vi "WLAN - TV - RW - UTIL - CenterFrequencyToChannelNumber_bc.vi"(0 "Center Frequency(Hz)":dbl=4940000000.0, 5 "Channel Bandwidth (Hz)":dbl=20000000.0) -> (4 "Coherced Channel Number":i32=188, 6 "Coherced Center Frequency (Hz)":dbl=5180000000.0)   [LabVIEW 2012]
doc: "Return channe numer according to channel bandwidth and center frequency."
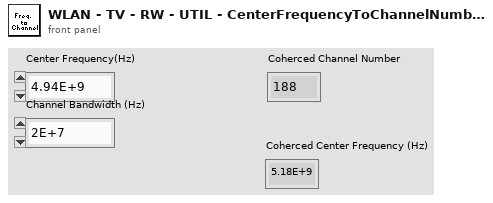
[diagram p1: front panel]
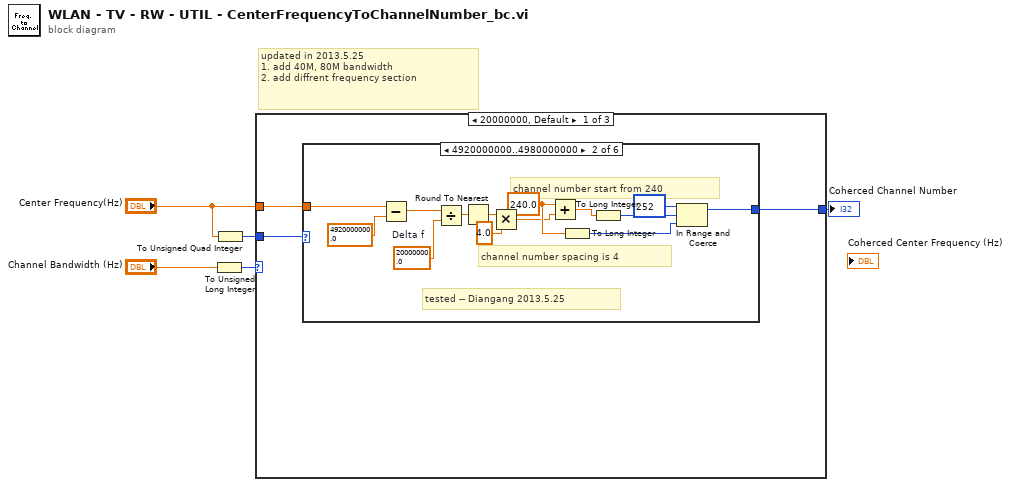
[diagram p0: block diagram]
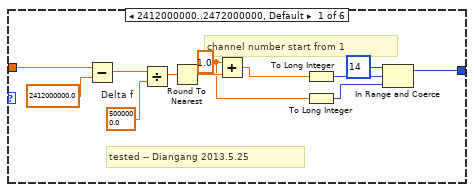
[diagram p2: hidden frame]
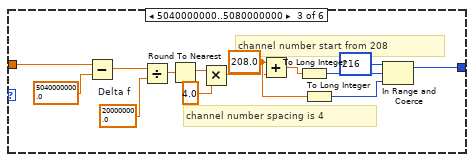
[diagram p3: hidden frame]
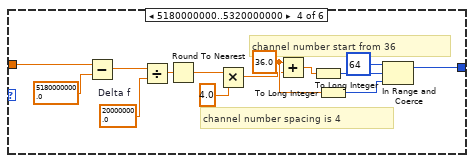
[diagram p4: hidden frame]
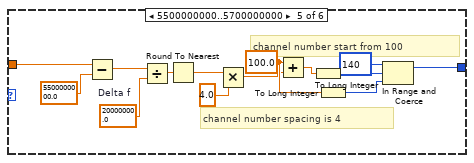
[diagram p5: hidden frame]
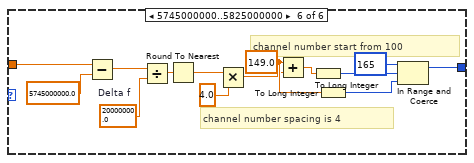
[diagram p6: hidden frame]
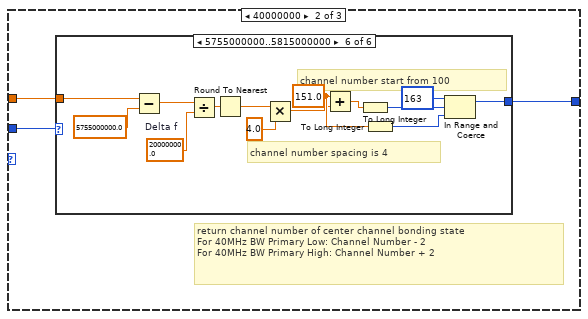
[diagram p7: hidden frame]
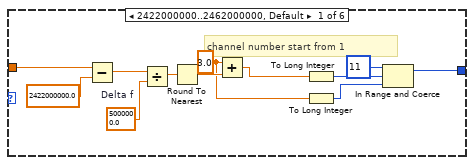
[diagram p8: hidden frame]
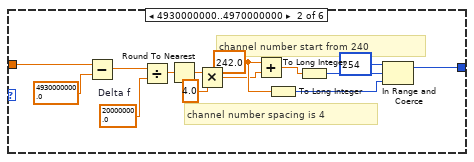
[diagram p9: hidden frame]
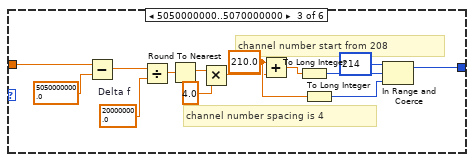
[diagram p10: hidden frame]
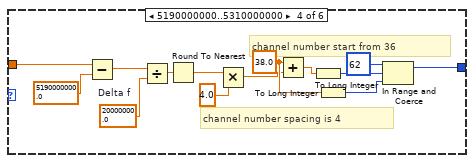
[diagram p11: hidden frame]
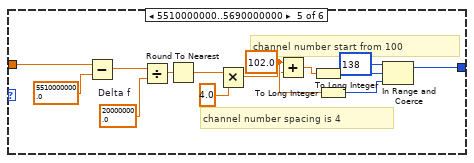
[diagram p12: hidden frame]
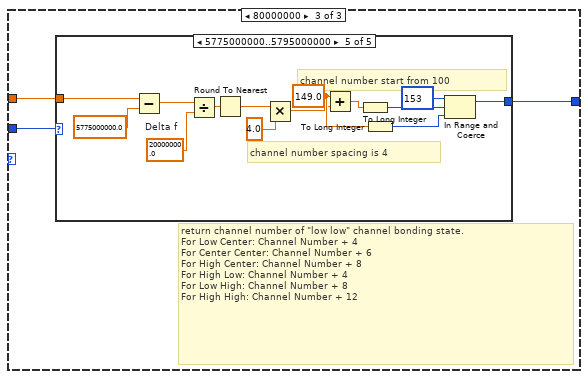
[diagram p13: hidden frame]
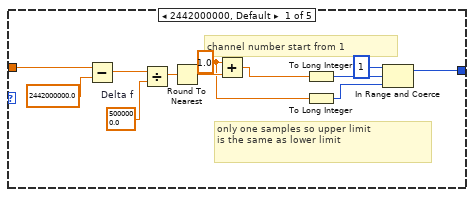
[diagram p14: hidden frame]
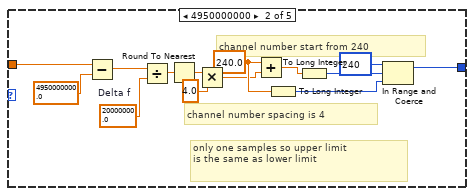
[diagram p15: hidden frame]
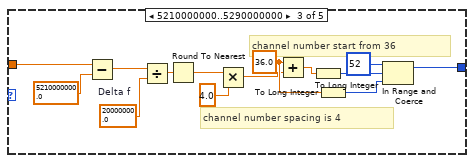
[diagram p16: hidden frame]
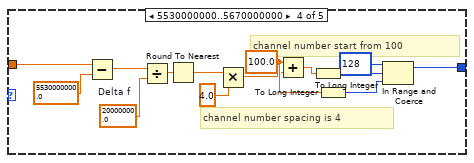
[diagram p17: hidden frame]
diagram:
  # "updated in 2013.5.25\n1. add 40M, 80M bandwidth\n2. add diffrent frequency section"
  n1 = To Unsigned Long Integer(number="Channel Bandwidth (Hz)") -> (unsigned 32bit integer=w4:u32)
  n2 = To Unsigned Quad Integer(1:"Center Frequency(Hz)") -> (0:w3:u64)
  n3 = case shown="20000000, Default" w4 {
    tunnel: w3 -> [w8 w93 w178]
    tunnel: "Center Frequency(Hz)" -> [w7 w92 w177]
    tunnel: [w6 w91 w176] -> w1
    frame 20000000, Default {
      n4 = case shown="4920000000..4980000000" w8 {
        tunnel: w7 -> [w17 w31 w45 w59 w73 w87]
        tunnel: [w14 w28 w42 w56 w70 w84] -> w6
        frame 2412000000..2472000000, Default {
          w9 = 1.0 ("x")
          w19 = 5000000.0  # Delta f
          # "channel number start from 1"
          # "tested -- Diangang 2013.5.25"
          n5 = Subtract(x=w17, y=2412000000.0) -> (x-y=w20:dbl)
          n6 = Divide(x=w20, y=w19) -> (x/y=w13:dbl)
          n7 = Round To Nearest(number=w13) -> (nearest integer value=w12:dbl)
          n8 = Add(x=w9, y=w12) -> (x+y=w11:dbl)
          n9 = To Long Integer(number=w11) -> (32bit integer=w15:i32)
          n10 = To Long Integer(number=w9) -> (32bit integer=w10:i32)
          n11 = In Range and Coerce(upper limit=14, x=w15, lower limit=w10) -> (coerced(x)=w14:i32)  [unwired: 1 out]
        }
        frame 4920000000..4980000000 {
          w24 = 240.0 ("x")
          w33 = 20000000.0  # Delta f
          # "tested -- Diangang 2013.5.25"
          # "channel number spacing is 4"
          # "channel number start from 240"
          n12 = Subtract(x=w31, y=4920000000.0) -> (x-y=w34:dbl)
          n13 = Divide(x=w34, y=w33) -> (x/y=w26:dbl)
          n14 = Round To Nearest(number=w26) -> (nearest integer value=w23:dbl)
          n15 = Multiply(x=w23, y=4.0) -> (x*y=w21:dbl)
          n16 = Add(x=w24, y=w21) -> (x+y=w27:dbl)
          n17 = To Long Integer(number=w24) -> (32bit integer=w25:i32)
          n18 = To Long Integer(number=w27) -> (32bit integer=w29:i32)
          n19 = In Range and Coerce(upper limit=252, x=w29, lower limit=w25) -> (coerced(x)=w28:i32)  [unwired: 1 out]
        }
        frame 5040000000..5080000000 {
          w39 = 208.0 ("x")
          w47 = 20000000.0  # Delta f
          # "channel number spacing is 4"
          # "channel number start from 208"
          n20 = Subtract(x=w45, y=5040000000.0) -> (x-y=w48:dbl)
          n21 = Divide(x=w48, y=w47) -> (x/y=w40:dbl)
          n22 = Round To Nearest(number=w40) -> (nearest integer value=w37:dbl)
          n23 = Multiply(x=w37, y=4.0) -> (x*y=w35:dbl)
          n24 = Add(x=w39, y=w35) -> (x+y=w41:dbl)
          n25 = To Long Integer(number=w41) -> (32bit integer=w43:i32)
          n26 = To Long Integer(number=w39) -> (32bit integer=w38:i32)
          n27 = In Range and Coerce(upper limit=216, x=w43, lower limit=w38) -> (coerced(x)=w42:i32)  [unwired: 1 out]
        }
        frame 5180000000..5320000000 {
          w53 = 36.0 ("x")
          w61 = 20000000.0  # Delta f
          # "channel number spacing is 4"
          # "channel number start from 36"
          n28 = Subtract(x=w59, y=5180000000.0) -> (x-y=w62:dbl)
          n29 = Divide(x=w62, y=w61) -> (x/y=w54:dbl)
          n30 = Round To Nearest(number=w54) -> (nearest integer value=w50:dbl)
          n31 = Multiply(x=w50, y=4.0) -> (x*y=w49:dbl)
          n32 = Add(x=w53, y=w49) -> (x+y=w55:dbl)
          n33 = To Long Integer(number=w55) -> (32bit integer=w57:i32)
          n34 = To Long Integer(number=w53) -> (32bit integer=w52:i32)
          n35 = In Range and Coerce(upper limit=64, x=w57, lower limit=w52) -> (coerced(x)=w56:i32)  [unwired: 1 out]
        }
        frame 5500000000..5700000000 {
          w67 = 100.0 ("x")
          w75 = 20000000.0  # Delta f
          # "channel number spacing is 4"
          # "channel number start from 100"
          n36 = Subtract(x=w73, y=5500000000.0) -> (x-y=w76:dbl)
          n37 = Divide(x=w76, y=w75) -> (x/y=w68:dbl)
          n38 = Round To Nearest(number=w68) -> (nearest integer value=w64:dbl)
          n39 = Multiply(x=w64, y=4.0) -> (x*y=w63:dbl)
          n40 = Add(x=w67, y=w63) -> (x+y=w69:dbl)
          n41 = To Long Integer(number=w69) -> (32bit integer=w71:i32)
          n42 = To Long Integer(number=w67) -> (32bit integer=w66:i32)
          n43 = In Range and Coerce(upper limit=140, x=w71, lower limit=w66) -> (coerced(x)=w70:i32)  [unwired: 1 out]
        }
        frame 5745000000..5825000000 {
          w81 = 149.0 ("x")
          w89 = 20000000.0  # Delta f
          # "channel number spacing is 4"
          # "channel number start from 100"
          n44 = Subtract(x=w87, y=5745000000.0) -> (x-y=w90:dbl)
          n45 = Divide(x=w90, y=w89) -> (x/y=w82:dbl)
          n46 = Round To Nearest(number=w82) -> (nearest integer value=w78:dbl)
          n47 = Multiply(x=w78, y=4.0) -> (x*y=w77:dbl)
          n48 = Add(x=w81, y=w77) -> (x+y=w83:dbl)
          n49 = To Long Integer(number=w83) -> (32bit integer=w85:i32)
          n50 = To Long Integer(number=w81) -> (32bit integer=w80:i32)
          n51 = In Range and Coerce(upper limit=165, x=w85, lower limit=w80) -> (coerced(x)=w84:i32)  [unwired: 1 out]
        }
      }
    }
    frame 40000000 {
      # "return channel number of center channel bonding state\nFor 40MHz BW Primary Low: Channel Number - 2\nFor 40MHz BW Primary High: Channel Number + 2"
      n52 = case shown="5755000000..5815000000" w93 {
        tunnel: w92 -> [w102 w116 w130 w144 w158 w172]
        tunnel: [w99 w113 w127 w141 w155 w169] -> w91
        frame 2422000000..2462000000, Default {
          w94 = 3.0 ("x")
          w104 = 5000000.0  # Delta f
          # "channel number start from 1"
          n53 = Subtract(x=w102, y=2422000000.0) -> (x-y=w105:dbl)
          n54 = Divide(x=w105, y=w104) -> (x/y=w98:dbl)
          n55 = Round To Nearest(number=w98) -> (nearest integer value=w97:dbl)
          n56 = Add(x=w94, y=w97) -> (x+y=w96:dbl)
          n57 = To Long Integer(number=w96) -> (32bit integer=w100:i32)
          n58 = To Long Integer(number=w94) -> (32bit integer=w95:i32)
          n59 = In Range and Coerce(upper limit=11, x=w100, lower limit=w95) -> (coerced(x)=w99:i32)  [unwired: 1 out]
        }
        frame 4930000000..4970000000 {
          w109 = 242.0 ("x")
          w118 = 20000000.0  # Delta f
          # "channel number spacing is 4"
          # "channel number start from 240"
          n60 = Subtract(x=w116, y=4930000000.0) -> (x-y=w119:dbl)
          n61 = Divide(x=w119, y=w118) -> (x/y=w111:dbl)
          n62 = Round To Nearest(number=w111) -> (nearest integer value=w108:dbl)
          n63 = Multiply(x=w108, y=4.0) -> (x*y=w106:dbl)
          n64 = Add(x=w109, y=w106) -> (x+y=w112:dbl)
          n65 = To Long Integer(number=w109) -> (32bit integer=w110:i32)
          n66 = To Long Integer(number=w112) -> (32bit integer=w114:i32)
          n67 = In Range and Coerce(upper limit=254, x=w114, lower limit=w110) -> (coerced(x)=w113:i32)  [unwired: 1 out]
        }
        frame 5050000000..5070000000 {
          w124 = 210.0 ("x")
          w132 = 20000000.0  # Delta f
          # "channel number spacing is 4"
          # "channel number start from 208"
          n68 = Subtract(x=w130, y=5050000000.0) -> (x-y=w133:dbl)
          n69 = Divide(x=w133, y=w132) -> (x/y=w125:dbl)
          n70 = Round To Nearest(number=w125) -> (nearest integer value=w122:dbl)
          n71 = Multiply(x=w122, y=4.0) -> (x*y=w120:dbl)
          n72 = Add(x=w124, y=w120) -> (x+y=w126:dbl)
          n73 = To Long Integer(number=w126) -> (32bit integer=w128:i32)
          n74 = To Long Integer(number=w124) -> (32bit integer=w123:i32)
          n75 = In Range and Coerce(upper limit=214, x=w128, lower limit=w123) -> (coerced(x)=w127:i32)  [unwired: 1 out]
        }
        frame 5190000000..5310000000 {
          w138 = 38.0 ("x")
          w146 = 20000000.0  # Delta f
          # "channel number spacing is 4"
          # "channel number start from 36"
          n76 = Subtract(x=w144, y=5190000000.0) -> (x-y=w147:dbl)
          n77 = Divide(x=w147, y=w146) -> (x/y=w139:dbl)
          n78 = Round To Nearest(number=w139) -> (nearest integer value=w135:dbl)
          n79 = Multiply(x=w135, y=4.0) -> (x*y=w134:dbl)
          n80 = Add(x=w138, y=w134) -> (x+y=w140:dbl)
          n81 = To Long Integer(number=w140) -> (32bit integer=w142:i32)
          n82 = To Long Integer(number=w138) -> (32bit integer=w137:i32)
          n83 = In Range and Coerce(upper limit=62, x=w142, lower limit=w137) -> (coerced(x)=w141:i32)  [unwired: 1 out]
        }
        frame 5510000000..5690000000 {
          w152 = 102.0 ("x")
          w160 = 20000000.0  # Delta f
          # "channel number spacing is 4"
          # "channel number start from 100"
          n84 = Subtract(x=w158, y=5510000000.0) -> (x-y=w161:dbl)
          n85 = Divide(x=w161, y=w160) -> (x/y=w153:dbl)
          n86 = Round To Nearest(number=w153) -> (nearest integer value=w149:dbl)
          n87 = Multiply(x=w149, y=4.0) -> (x*y=w148:dbl)
          n88 = Add(x=w152, y=w148) -> (x+y=w154:dbl)
          n89 = To Long Integer(number=w154) -> (32bit integer=w156:i32)
          n90 = To Long Integer(number=w152) -> (32bit integer=w151:i32)
          n91 = In Range and Coerce(upper limit=138, x=w156, lower limit=w151) -> (coerced(x)=w155:i32)  [unwired: 1 out]
        }
        frame 5755000000..5815000000 {
          w166 = 151.0 ("x")
          w174 = 20000000.0  # Delta f
          # "channel number spacing is 4"
          # "channel number start from 100"
          n92 = Subtract(x=w172, y=5755000000.0) -> (x-y=w175:dbl)
          n93 = Divide(x=w175, y=w174) -> (x/y=w167:dbl)
          n94 = Round To Nearest(number=w167) -> (nearest integer value=w163:dbl)
          n95 = Multiply(x=w163, y=4.0) -> (x*y=w162:dbl)
          n96 = Add(x=w166, y=w162) -> (x+y=w168:dbl)
          n97 = To Long Integer(number=w168) -> (32bit integer=w170:i32)
          n98 = To Long Integer(number=w166) -> (32bit integer=w165:i32)
          n99 = In Range and Coerce(upper limit=163, x=w170, lower limit=w165) -> (coerced(x)=w169:i32)  [unwired: 1 out]
        }
      }
    }
    frame 80000000 {
      # "return channel number of \"low low\" channel bonding state.\nFor Low Center: Channel Number + 4\nFor Center Center: Channel Number + 6\nFor High Center: Channel Number + 8\nFor High Low: Channel Number + 4\nFor Low High: Channel Number + 8\nFor High High: Channel Number + 12"
      n100 = case shown="5775000000..5795000000" w178 {
        tunnel: w177 -> [w187 w201 w215 w229 w243]
        tunnel: [w184 w198 w212 w226 w240] -> w176
        frame 2442000000, Default {
          w179 = 1.0 ("x")
          w189 = 5000000.0  # Delta f
          # "only one samples so upper limit\nis the same as lower limit"
          # "channel number start from 1"
          n101 = Subtract(x=w187, y=2442000000.0) -> (x-y=w190:dbl)
          n102 = Divide(x=w190, y=w189) -> (x/y=w183:dbl)
          n103 = Round To Nearest(number=w183) -> (nearest integer value=w182:dbl)
          n104 = Add(x=w179, y=w182) -> (x+y=w181:dbl)
          n105 = To Long Integer(number=w181) -> (32bit integer=w185:i32)
          n106 = To Long Integer(number=w179) -> (32bit integer=w180:i32)
          n107 = In Range and Coerce(upper limit=1, x=w185, lower limit=w180) -> (coerced(x)=w184:i32)  [unwired: 1 out]
        }
        frame 4950000000 {
          w194 = 240.0 ("x")
          w203 = 20000000.0  # Delta f
          # "only one samples so upper limit\nis the same as lower limit"
          # "channel number spacing is 4"
          # "channel number start from 240"
          n108 = Subtract(x=w201, y=4950000000.0) -> (x-y=w204:dbl)
          n109 = Divide(x=w204, y=w203) -> (x/y=w196:dbl)
          n110 = Round To Nearest(number=w196) -> (nearest integer value=w193:dbl)
          n111 = Multiply(x=w193, y=4.0) -> (x*y=w191:dbl)
          n112 = Add(x=w194, y=w191) -> (x+y=w197:dbl)
          n113 = To Long Integer(number=w194) -> (32bit integer=w195:i32)
          n114 = To Long Integer(number=w197) -> (32bit integer=w199:i32)
          n115 = In Range and Coerce(upper limit=240, x=w199, lower limit=w195) -> (coerced(x)=w198:i32)  [unwired: 1 out]
        }
        frame 5210000000..5290000000 {
          w209 = 36.0 ("x")
          w217 = 20000000.0  # Delta f
          # "channel number spacing is 4"
          # "channel number start from 36"
          n116 = Subtract(x=w215, y=5210000000.0) -> (x-y=w218:dbl)
          n117 = Divide(x=w218, y=w217) -> (x/y=w210:dbl)
          n118 = Round To Nearest(number=w210) -> (nearest integer value=w206:dbl)
          n119 = Multiply(x=w206, y=4.0) -> (x*y=w205:dbl)
          n120 = Add(x=w209, y=w205) -> (x+y=w211:dbl)
          n121 = To Long Integer(number=w211) -> (32bit integer=w213:i32)
          n122 = To Long Integer(number=w209) -> (32bit integer=w208:i32)
          n123 = In Range and Coerce(upper limit=52, x=w213, lower limit=w208) -> (coerced(x)=w212:i32)  [unwired: 1 out]
        }
        frame 5530000000..5670000000 {
          w223 = 100.0 ("x")
          w231 = 20000000.0  # Delta f
          # "channel number spacing is 4"
          # "channel number start from 100"
          n124 = Subtract(x=w229, y=5530000000.0) -> (x-y=w232:dbl)
          n125 = Divide(x=w232, y=w231) -> (x/y=w224:dbl)
          n126 = Round To Nearest(number=w224) -> (nearest integer value=w220:dbl)
          n127 = Multiply(x=w220, y=4.0) -> (x*y=w219:dbl)
          n128 = Add(x=w223, y=w219) -> (x+y=w225:dbl)
          n129 = To Long Integer(number=w225) -> (32bit integer=w227:i32)
          n130 = To Long Integer(number=w223) -> (32bit integer=w222:i32)
          n131 = In Range and Coerce(upper limit=128, x=w227, lower limit=w222) -> (coerced(x)=w226:i32)  [unwired: 1 out]
        }
        frame 5775000000..5795000000 {
          w237 = 149.0 ("x")
          w245 = 20000000.0  # Delta f
          # "channel number spacing is 4"
          # "channel number start from 100"
          n132 = Subtract(x=w243, y=5775000000.0) -> (x-y=w246:dbl)
          n133 = Divide(x=w246, y=w245) -> (x/y=w238:dbl)
          n134 = Round To Nearest(number=w238) -> (nearest integer value=w234:dbl)
          n135 = Multiply(x=w234, y=4.0) -> (x*y=w233:dbl)
          n136 = Add(x=w237, y=w233) -> (x+y=w239:dbl)
          n137 = To Long Integer(number=w239) -> (32bit integer=w241:i32)
          n138 = To Long Integer(number=w237) -> (32bit integer=w236:i32)
          n139 = In Range and Coerce(upper limit=153, x=w241, lower limit=w236) -> (coerced(x)=w240:i32)  [unwired: 1 out]
        }
      }
    }
  }
  "Coherced Channel Number" <- w1
